vi "Agilent DMM Read Blank Screen.vi"(8 "error in (no error)":errorcluster, 11 "VISA Resource Name":refnum<visa-resource-name>) -> (0 "error out":errorcluster, 2 "Blank Screen":bool, 3 "dup VISA Resource Name":refnum<visa-resource-name>)   [LabVIEW 2011]
doc: "This VI for the HP 8753 is used to read the sweep type.\n\n0 LINEAR FREQ\n1 LOG FREQ\n2 LIST FREQ\n3 CW TIME\n4 POWER SWEEP"
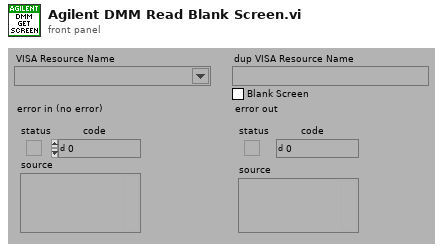
[diagram p1: front panel]
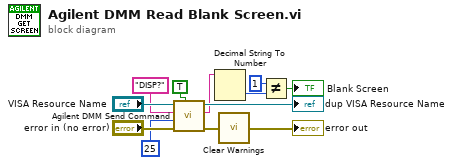
[diagram p0: block diagram]
diagram:
  n1 = call "Agilent DMM Send Command.vi"("Read? (F)"=TRUE, "error in (no error)"="error in (no error)", "Byte Count"=u32 25 ("byte count"), "Command"="DISP?" ("write buffer"), "VISA Resource Name"="VISA Resource Name") -> ("error out"=w5:errorcluster, "Data Read"=w3:string, "dup VISA Resource Name"=→"dup VISA Resource Name":refnum<visa-resource-name>)  [unwired: 4 out]
  n2 = Decimal String To Number(string=w3) -> (number=w7:i32)  [unwired: 3 out]
  n3 = call "Clear Warnings.vi"("error in (no error)"=w5) -> ("error out"=→"error out":errorcluster)
  n4 = Not Equal?(x=1, y=w7) -> (x != y?=→"Blank Screen":bool)
